vi "ws_www template global keys.vi"(6 "Current User":T1, 7 "httpRequestID":u32, 8 "error in (no error)":errorcluster, 10 "Template Keys In (empty)":T2, 11 "DB Connection Ref":T3) -> (0 "error out":errorcluster, 2 "new Template Keys":T2, 3 "dup DB Connection Ref":T3)   [LabVIEW 2011]
uses:
  SI.LIB/ODBC/SQL Controls/Connection Refnum.ctl
  <vilib>/addons/internet/utils/keyedarr.llb/Keyed Array.ctl
  server/database/Users/User Record.ctl
  <vilib>/wsapi/NI_WebServices.lvlib
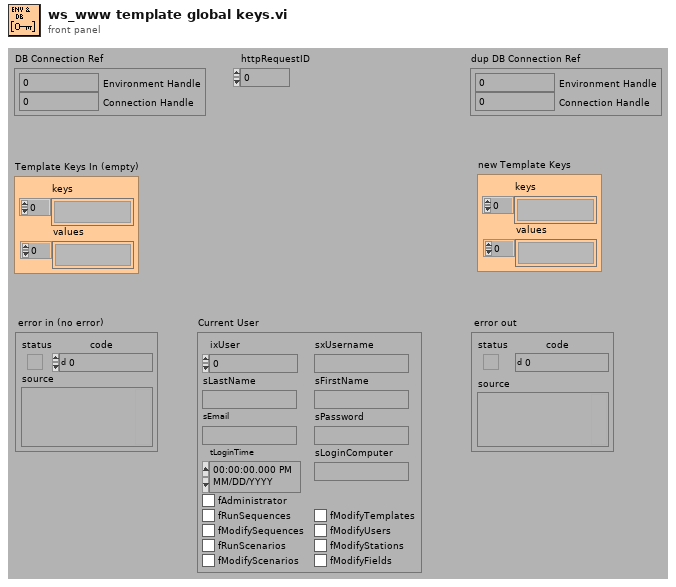
[diagram p1: front panel]
types:
  T1 = typedef "User Record.ctl" = cluster{"ixUser":i32, "sxUsername":string, "sLastName":string, "sFirstName":string, "sEmail":string, "sPassword":string, "tLoginTime":timestamp, "sLoginComputer":string, "fAdministrator":bool, "fRunSequences":bool, "fModifySequences":bool, "fRunScenarios":bool, "fModifyScenarios":bool, "fModifyTemplates":bool, "fModifyUsers":bool, "fModifyStations":bool, "fModifyFields":bool}
  T2 = typedef "Keyed Array.ctl" = cluster{"keys":string[], "values":string[]}
  T3 = typedef "Connection Refnum.ctl" = cluster{"Environment Handle":i32, "Connection Handle":i32}
  T4 = typedef "OGAB Version.ctl" = cluster{"Version":string, "Build Number":u32, "Build Date/Time":dbl}
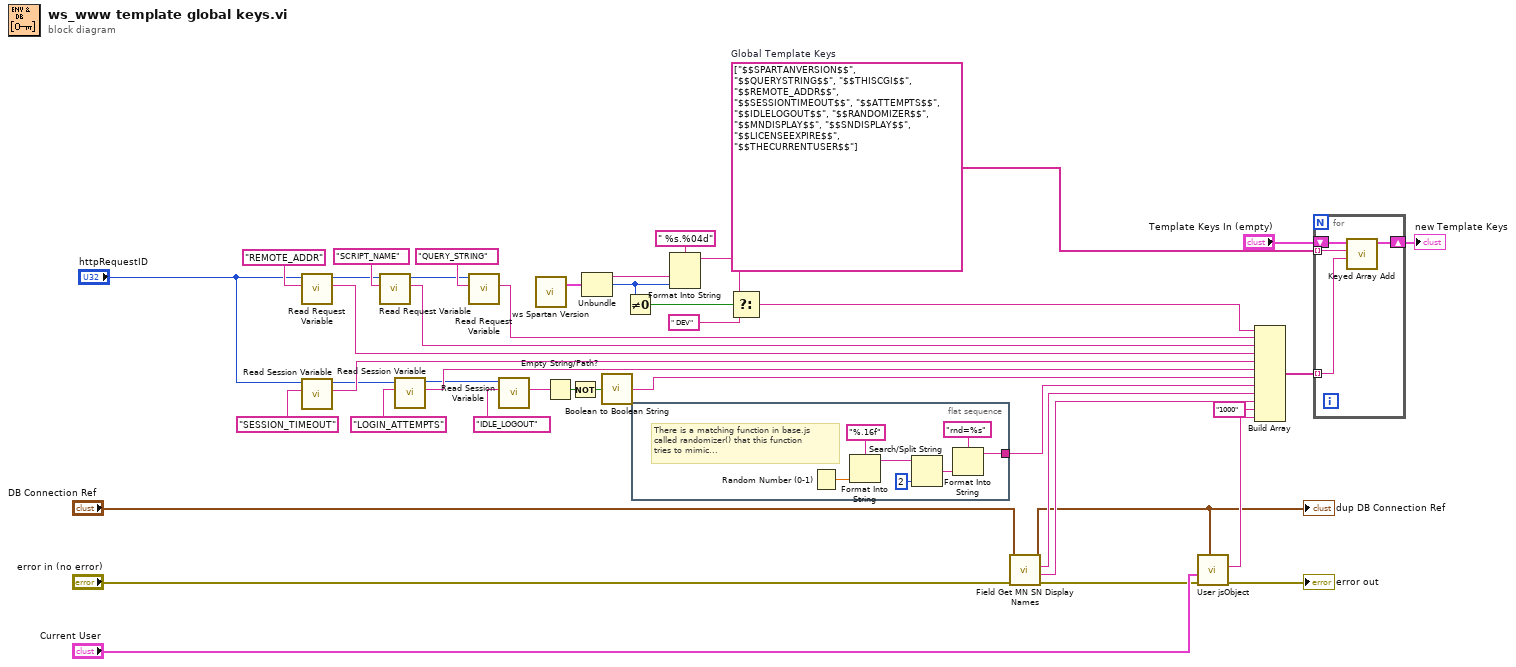
[diagram p0: block diagram]
diagram:
  w41 = string[] ["$$SPARTANVERSION$$", "$$QUERYSTRING$$", "$$THISCGI$$", "$$REMOTE_ADDR$$", "$$SESSIONTIMEOUT$$", "$$ATTEMPTS$$", "$$IDLELOGOUT$$", "$$RANDOMIZER$$", "$$MNDISPLAY$$", "$$SNDISPLAY$$", "$$LICENSEEXPIRE$$", "$$THECURRENTUSER$$"]  # Global Template Keys
  n1 = call <vilib>:"Read Request Variable.vi"("variable name"="REMOTE_ADDR", "httpRequestID"="httpRequestID") -> ("value"=w17:string, "httpRequestID out"=w19:u32)  [unwired: 7 in, 1 out]
  n2 = call <vilib>:"Read Session Variable.vi"("key"="SESSION_TIMEOUT", "httpRequestID"="httpRequestID") -> ("value"=w15:string, "httpRequestID out"=w13:u32)  [unwired: 7 in, 1 out]
  n3 = call <vilib>:"Read Request Variable.vi"("variable name"="SCRIPT_NAME" ("name"), "httpRequestID"=w19) -> ("value"=w20:string, "httpRequestID out"=w21:u32)  [unwired: 7 in, 1 out]
  n4 = call <vilib>:"Read Session Variable.vi"("key"="LOGIN_ATTEMPTS", "httpRequestID"=w13) -> ("value"=w11:string, "httpRequestID out"=w10:u32)  [unwired: 7 in, 1 out]
  n5 = call <vilib>:"Read Request Variable.vi"("variable name"="QUERY_STRING" ("name"), "httpRequestID"=w21) -> ("value"=w23:string)  [unwired: 7 in, 2 out]
  n6 = call <vilib>:"Read Session Variable.vi"("key"="IDLE_LOGOUT", "httpRequestID"=w10) -> ("value"=w8:string)  [unwired: 7 in, 2 out]
  n7 = call "ws Spartan Version.vi"() -> ("Version"=w4:T4)  [unwired: 3 in]
  n8 = Empty String/Path?(string/path=w8) -> (empty?=w7:bool)
  n9 = Not(x=w7) -> (.not. x?=w6:bool)
  n10 = Unbundle(w4) -> ("Version"=w29:string, "Build Number"=w33:u32)  [unwired: 1 out]
  n11 = call "Boolean to Boolean String.vi"("Boolean"=w6) -> ("Boolean string"=w5:string)  [unwired: 1 in]
  n12 = Not Equal To 0?(x=w33) -> (x != 0?=w30:bool)
  n13 = flat-sequence {
    tunnel: [w44] -> w28
    frame #0 {
      # "There is a matching function in base.js\ncalled randomizer() that this function\ntries to mimic..."
      n14 = Random Number (0-1)() -> (number: 0 to 1=w50:dbl)
      n15 = Format Into String(format string="%.16f", w50) -> (resulting string=w45:string)  [unwired: 2 in, 1 out]
      n16 = Search/Split String(string=w45, offset (0)=2) -> (match + rest of string=w47:string)  [unwired: 3 out]
      n17 = Format Into String(format string="rnd=%s", w47) -> (resulting string=w44:string)  [unwired: 2 in, 1 out]
    }
  }
  n18 = Format Into String(format string=" %s.%04d", w29, w33) -> (resulting string=w26:string)  [unwired: 2 in, 1 out]
  n19 = Select(t=w26, s=w30, f=" DEV") -> (s? t:f=w31:string)
  n20 = call "Field Get MN SN Display Names.vi"("error in (no error)"="error in (no error)", "Connection Refnum"="DB Connection Ref") -> ("error out"=w2:errorcluster, "Serial Number Display Name"=w39:string, "Model Number Display Name"=w40:string, "Connection Refnum"=w3:T3)  [unwired: 6 out]
  "dup DB Connection Ref" <- w3
  n21 = call "User jsObject.vi"("DB Connection Ref"=w3, "error in (no error)"=w2, "User Record (empty)"="Current User") -> ("error out"=→"error out":errorcluster, "User Literal Object"=w27:string)  [unwired: 2 in, 5 out]
  n22 = Build Array(w31, w23, w20, w17, w15, w11, w5, w28, w40, w39, "1000" ("element"), w27) -> (w38:string[])
  n23 = for {
    shift-right: [w53] -> w36
    shift-left: "Template Keys In (empty)" -> [w54]
    tunnel: w41 -> [w52] mode=indexing
    tunnel: w38 -> [w51] mode=indexing
    n24 = call <vilib>:"Keyed Array Add.vi"("value"=w51, "key"=w52, "array in"=w54) -> ("array out"=w53:T2)  [unwired: 2 in, 2 out]
  }
  "new Template Keys" <- w36
